vi "Keithley 2002 Burst Mode.vi"(0 "GPIB address":string="16", 1 "source (imm:1)":u16(ring)=1 items=["hold", "immediate", "timer", "manual", "bus", "trigger link", "external"], 2 "function (Vdc:1)":u16(ring)=1 items=["ac voltage", "dc voltage", "2-wire resistance", "ac current", "dc current"], 3 "error in":T1, 4 "# of readings":dbl=100.0 min=2.0 max=3280.0 step=1.0) -> (5 "measurements":dbl[](array[numeric]) format="%.6e", 6 "error out":T1)   [LabVIEW 2020]
doc: "This VI is used to take burst measurements. These are fast readings that can only be made with certain functions selected.\n\nNote: The instrument will display a message saying \"Burst\n Mode Aborted\". This message should be ignored.\n The VI is merely taking the instrument out of the Burst\n Mode after the measurements have been taken.\n\nThe measurements are optimized for the fastest possible reading, and then when the operation is complete, the original configuration goes back into effect.\n\nThe readings do not include time stamp, channel number, or any other information other than the actual value."
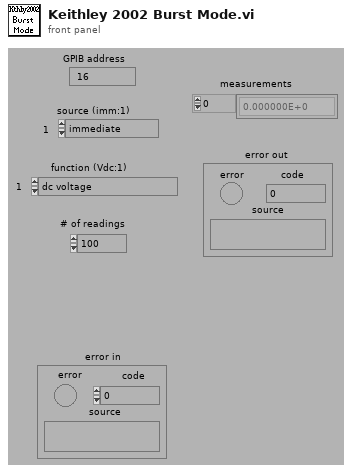
[diagram p1: front panel]
types:
  T1 = cluster{"error":bool, "code":i32, "source":string}
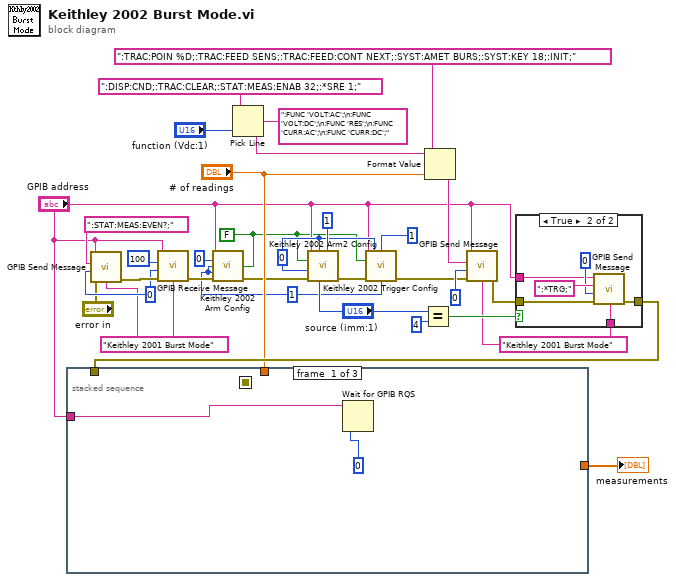
[diagram p0: block diagram]
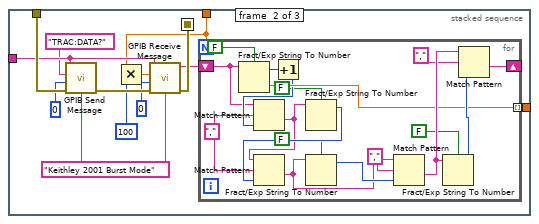
[diagram p3: hidden frame]
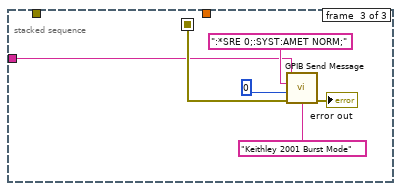
[diagram p4: hidden frame]
diagram:
  w21 = "Keithley 2001 Burst Mode"
  w27 = 0
  w5 = 0
  w3 = FALSE
  w1 = 1
  w23 = "Keithley 2001 Burst Mode"
  n1 = call "GPIB Send Message.vi"("address string"="GPIB address", "write buffer"=":STAT:MEAS:EVEN?;", "source"=w21, "write mode (set END:0)"=w27, "error in"="error in") -> ("error out"=w30:T1)  [unwired: 2 in, 2 out]
  n2 = call "GPIB Receive Message.vi"("address string"="GPIB address", "byte count"=100, "source"=w21, "read mode"=w27, "error in"=w30) -> ("error out"=w10:T1)  [unwired: 2 in, 2 out]
  n3 = call "Keithley 2002 Arm Config.vi"("GPIB address"="GPIB address", "count (set:0)"=0, "count value"=w1, "direction"=w3, "source (imm:1)"=w1, "error in"=w10) -> ("error out"=w9:T1)  [unwired: 9 in]
  n4 = Pick Line(string ("")=":DISP:CND;:TRAC:CLEAR;:STAT:MEAS:ENAB 32;:*SRE 1;", multi-line string=":FUNC 'VOLT:AC';\n:FUNC 'VOLT:DC';\n:FUNC 'RES';\n:FUNC 'CURR:AC';\n:FUNC 'CURR:DC';", line index="function (Vdc:1)") -> (output string=w14:string)
  n5 = call "Keithley 2002 Arm2 Config.vi"("count value"=1, "source (imm:1)"="source (imm:1)", "count (set:0)"=w5, "error in"=w9, "delay (secs)"=w5, "direction"=w3, "GPIB address"="GPIB address") -> ("error out"=w8:T1)  [unwired: 4 in]
  n6 = call "Keithley 2002 Trigger Config.vi"("GPIB address"="GPIB address", "count (set:0)"=w5, "count value"=1, "direction"=w3, "error in"=w8, "timer value (secs)"=w1) -> ("error out"=w11:T1)  [unwired: 9 in]
  n7 = Equal?(x="source (imm:1)", y=4) -> (x = y?=w24:bool)
  n8 = Format Value(string ("")=w14, format string=":TRAC:POIN %D;:TRAC:FEED SENS;:TRAC:FEED:CONT NEXT;:SYST:AMET BURS;:SYST:KEY 18;:INIT;", value (0)="# of readings") -> (output string=w15:string)
  n9 = call "GPIB Send Message.vi"("address string"="GPIB address", "write buffer"=w15, "source"=w23, "write mode (set END:0)"=0, "error in"=w11) -> ("error out"=w25:T1)  [unwired: 2 in, 2 out]
  n10 = case shown="True" w24 {
    tunnel: [w33 w35] -> w22
    tunnel: w23 -> [_ w34]
    tunnel: "GPIB address" -> [_ w36]
    tunnel: w25 -> [w33 w37]
    frame False {
    }
    frame True {
      n11 = call "GPIB Send Message.vi"("address string"=w36, "write buffer"=":*TRG;", "source"=w34, "write mode (set END:0)"=0, "error in"=w37) -> ("error out"=w35:T1)  [unwired: 2 in, 2 out]
    }
  }
  n12 = stacked-sequence {
    seq-local: [_ w54 _] -> [_ _ w76]
    tunnel: "# of readings" -> [_ w42 _]
    tunnel: "GPIB address" -> [w40 w51 w75]
    tunnel: w22 -> [_ w53 _]
    tunnel: [_ w43 _] -> w12
    frame #0 {
      n13 = Wait for GPIB RQS(3:0, 4:w40) -> ()  [unwired: 1 in, 2 out]
    }
    frame #1 {
      w50 = "Keithley 2001 Burst Mode"
      n14 = call "GPIB Send Message.vi"("address string"=w51, "write buffer"="TRAC:DATA?", "source"=w50, "write mode (set END:0)"=0, "error in"=w53) -> ("error out"=w52:T1)  [unwired: 2 in, 2 out]
      n15 = Multiply(x=w42, y=100) -> (x*y=w45:dbl)
      n16 = call "GPIB Receive Message.vi"("address string"=w51, "byte count"=w45, "source"=w50, "read mode"=0, "error in"=w52) -> ("read buffer"=w44:string, "error out"=w54:T1)  [unwired: 2 in, 1 out]
      n17 = for {
        N: w42 -> [_]
        shift-right: [w63] -> _
        shift-left: w44 -> [w59]
        tunnel: [w61] -> w43 mode=indexing
        w68 = ","
        n18 = Fract/Exp String To Number(use system decimal point (T)=FALSE, string=w59) -> (offset past number=w62:i32, number=w61:dbl)  [unwired: 2 in]
        n19 = Increment(x=w62) -> (x+1=w60:i32)
        n20 = Match Pattern(string=w59, regular expression=w68, offset (0)=w60) -> (after substring=w71:string)  [unwired: 3 out]
        n21 = Fract/Exp String To Number(use system decimal point (T)=FALSE, string=w71) -> (offset past number=w72:i32)  [unwired: 2 in, 1 out]
        n22 = Match Pattern(string=w71, regular expression=w68, offset (0)=w72) -> (after substring=w69:string)  [unwired: 3 out]
        n23 = Fract/Exp String To Number(use system decimal point (T)=FALSE, string=w69) -> (offset past number=w70:i32)  [unwired: 2 in, 1 out]
        n24 = Match Pattern(string=w69, regular expression=",", offset (0)=w70) -> (after substring=w66:string)  [unwired: 3 out]
        n25 = Fract/Exp String To Number(use system decimal point (T)=FALSE, string=w66) -> (offset past number=w65:i32)  [unwired: 2 in, 1 out]
        n26 = Match Pattern(string=w66, regular expression=",", offset (0)=w65) -> (after substring=w63:string)  [unwired: 3 out]
      }
    }
    frame #2 {
      n27 = call "GPIB Send Message.vi"("address string"=w75, "write buffer"=":*SRE 0;:SYST:AMET NORM;", "source"="Keithley 2001 Burst Mode", "write mode (set END:0)"=0, "error in"=w76) -> ("error out"=→"error out":T1)  [unwired: 2 in, 2 out]
    }
  }
  "measurements" <- w12
